vi "GetResponse00.vi"(2 "delay before read (ms)":u32=500, 3 "input":string, 4 "error in (no error)":errorcluster, 5 "VISA resource name":refnum<visa-resource-name>) -> (0 "error out":errorcluster, 1 "VISA resource name out":refnum<visa-resource-name>)   [LabVIEW 2011]
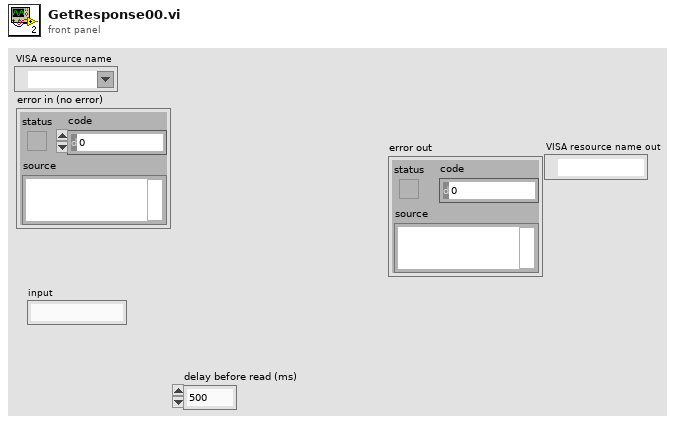
[diagram p1: front panel]
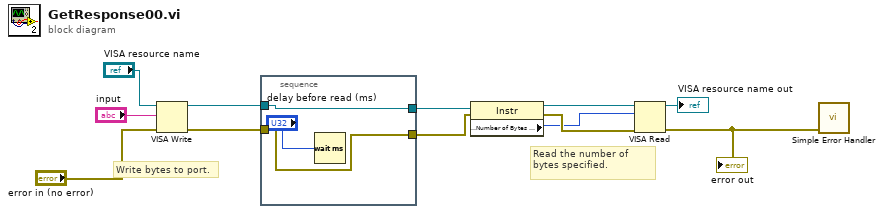
[diagram p0: block diagram]
diagram:
  # "Write bytes to port."
  # "Read the number of bytes specified."
  n1 = VISA Write(VISA resource name="VISA resource name", write buffer="input", error in (no error)="error in (no error)") -> (VISA resource name out=w9:refnum<visa-resource-name>, error out=w8:errorcluster)  [unwired: 1 out]
  n2 = stacked-sequence {
    tunnel: w9 -> [w14]
    tunnel: w8 -> [w13]
    tunnel: [w14] -> w7
    tunnel: [w13] -> w6
    frame #0 {
      n3 = Wait (ms)(milliseconds to wait="delay before read (ms)") -> ()  [unwired: 1 out]
    }
  }
  n4 = property class="Instr"(reference=w7, error in=w6) -> (reference out=w12:refnum<visa-resource-name>, error out=w11:errorcluster, "Serial Settings:Number of Bytes at Serial Port"=w10:u32)
  n5 = VISA Read(VISA resource name=w12, byte count=w10, error in (no error)=w11) -> (VISA resource name out=→"VISA resource name out":refnum<visa-resource-name>, error out=w5:errorcluster)  [unwired: 2 out]
  "error out" <- w5
  n6 = call <vilib>:"Simple Error Handler.vi"("error in (no error)"=w5) -> ()  [unwired: 1 in, 8 out]
